vi "Login.vi"() -> ()   [LabVIEW 2020]
uses:
  Global1.vi
panel:
  in  "联机模式":enum16{"单机", "追溯"}(ring)
  in  "密码":string
  in  "账号":string
  in  "确定":bool
  # "锁卡及精密定位圈压装台"
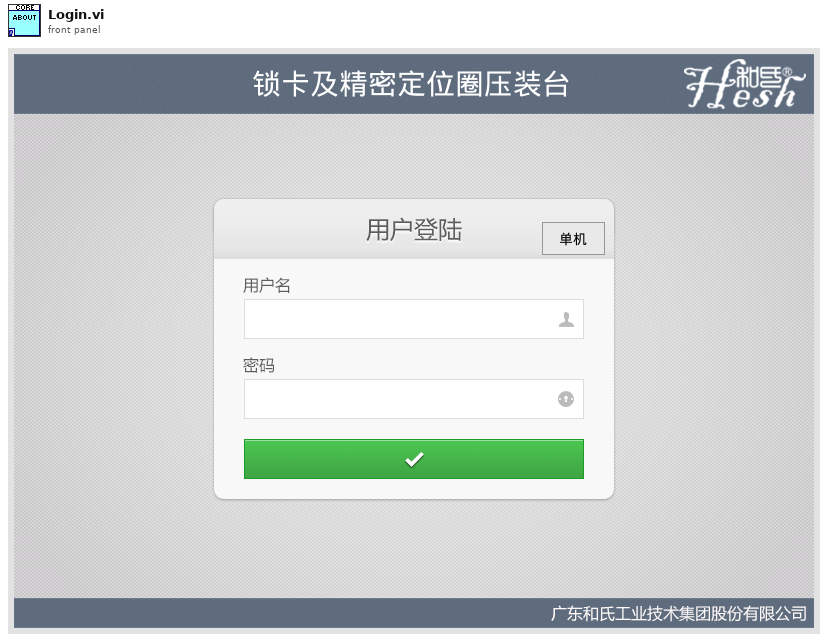
[diagram p1: front panel]
types:
  T1 = enum32{"Invalid", "Standard", "Closed", "Hidden", "Minimized", "Maximized"}
  T2 = cluster{"data[0]":string, "data[1]":string, "data[2]":string, "data[3]":string}
  T3 = typedef "eventvkey.ctl" = enum16{"ASCII", "Enter", "Return", "Shift", "Ctrl", "Alt", "Cmd", "Opt", "Caps", "NumLock", "Clear", "Break", "Up", "Down", "Left", "Right", "Insert", "Delete", "Home", "End", "PageUp", "PageDown", "Escape", "Help", "Pause", "ScrollLock", "F1", "F2", "F3", "F4", "F5", "F6", "F7", "F8", "F9", "F10", "F11", "F12", "F13", "F14", "F15", "F16", "F17", "F18", "F19", "F20", "F21", "F22", "F23", "F24", "Play", "VolumeUp", "VolumeDown", "Mute", "Two Byte Char"}
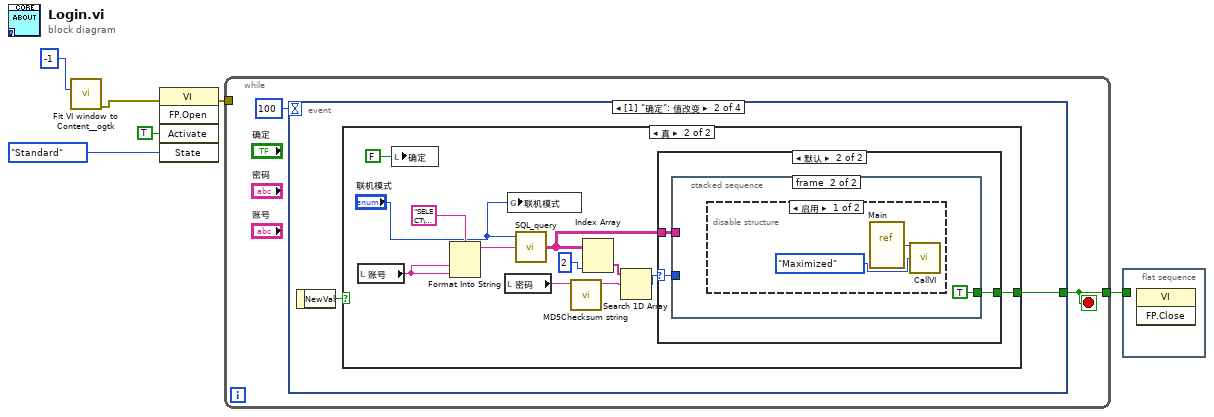
[diagram p0: block diagram]
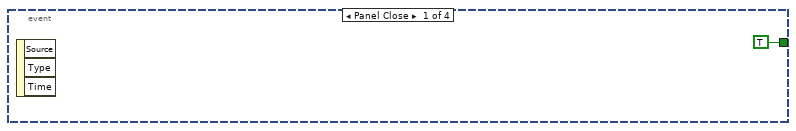
[diagram p2: hidden frame]
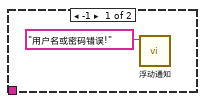
[diagram p4: hidden frame]
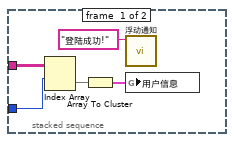
[diagram p5: hidden frame]
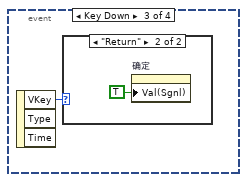
[diagram p7: hidden frame]
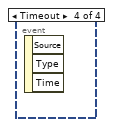
[diagram p9: hidden frame]
diagram:
  n1 = call <userlib>:"Fit VI window to Content__ogtk.vi"("border spacing (2 px)"=-1) -> ("error out"=w1:errorcluster)  [unwired: 5 in, 1 out]
  n2 = invoke class="VI" method="FP.Open"(error in=w1, "Activate"=TRUE ("Activate?"), "State"=T1."Standard") -> (error out=w3:errorcluster)  [unwired: 2 in, 4 out]
  n3 = while {
    tunnel: [w8] -> w6
    tunnel: w3 -> [_]
    stop <- w8 stop-if-true
    n4 = event shown="[1] \"确定\": 值改变" {
      selector: _ -> [_ _ _ _]
      dyn-events: _ -> [_ _ _ _]
      timeout: 100 -> [_ _ _ _]
      tunnel: [TRUE w10 _ _] -> w8
      event Panel Close {
        n5 = event-data() -> ()  [unwired: 4 out]
      }
      event "确定": Value Change {
        n6 = event-data() -> ("NewVal"=w11:bool)  [unwired: 1 out]
        n7 = case shown="真" w11 {
          tunnel: [_ w14] -> w10
          frame False {
          }
          frame True {
            n8 = local read "账号"() -> (w20:string)
            n9 = local write "确定"(FALSE ("确定")) -> ()
            n10 = Format Into String(format string="SELECT\ndbo.[User].USER_EMPLOYEE_ID,\ndbo.[User].USER_NAME,\ndbo.[User].USER_PASSWD,\ndbo.[User].USER_PERMIT\n\nFROM\ndbo.[User]\nWHERE\ndbo.[User].USER_NAME = '%s' \nOR\ndbo.[User].USER_EMPLOYEE_ID = '%s'\n" ("格式字符串"), w20, w20) -> (resulting string=w17:string)  [unwired: 2 in, 1 out]
            n11 = local read "密码"() -> (w21:string)
            n12 = global write "Global1.vi" "联机模式"("联机模式") -> ()
            n13 = call "SQL_query.vi"("SQL query"=w17, "联机模式"="联机模式") -> ("data"=w15:string[][])  [unwired: 1 in, 2 out]
            n14 = call <vilib>:"MD5Checksum string.vi"("Message String"=w21) -> ("MD5 message-digest"=w22:string)  [unwired: 10 in]
            n15 = Index Array(array=w15, index (col)=2 ("禁用的索引 (列)")) -> (element=w19:string[])  [unwired: 1 in]
            n16 = Search 1D Array(1D array=w19, element=w22) -> (index of element=w16:i32)  [unwired: 1 in]
            n17 = case shown="默认" w16 {
              selector: w16 -> [_ w26]
              tunnel: w15 -> [_ w27]
              tunnel: [_ w25] -> w14
              frame -1 {
                n18 = call "浮动通知.vi"("通知内容"="用户名或密码错误!") -> ()  [unwired: 11 in]
              }
              frame Default {
                n19 = stacked-sequence {
                  tunnel: w27 -> [w32 _]
                  tunnel: w26 -> [w31 _]
                  tunnel: [_ TRUE] -> w25
                  frame #0 {
                    n20 = Index Array(array=w32, index (row)=w31) -> (element=w29:string[])  [unwired: 1 in]
                    n21 = Array To Cluster(array=w29) -> (cluster=w28:T2)
                    n22 = call "浮动通知.vi"("通知内容"="登陆成功!") -> ()  [unwired: 11 in]
                    n23 = global write "Global1.vi" "用户信息"(w28) -> ()
                  }
                  frame #1 {
                    n24 = disable-structure shown="启用" {
                      frame Enabled {
                        n25 = vi-ref "Main.vi"() -> (w35:refnum<vi>)
                        n26 = call "CallVI.vi"("VI引用"=w35, "状态"=T1."Maximized") -> ()  [unwired: 11 in, 3 out]
                      }
                      frame Disabled {
                      }
                    }
                  }
                }
              }
            }
          }
        }
      }
      event Key Down {
        n27 = event-data() -> ("VKey"=w36:T3)  [unwired: 3 out]
        n28 = case shown="\"Return\"" w36 {
          frame Default {
          }
          frame "Return" {
            n29 = property on="确定" class="Bool (严格)"("Val(Sgnl)"=TRUE ("值(信号)")) -> ()  [unwired: 2 in, 2 out]
          }
        }
      }
      event Timeout {
        n30 = event-data() -> ()  [unwired: 4 out]
      }
    }
  }
  n31 = flat-sequence {
    tunnel: w6 -> [_]
    frame #0 {
      n32 = invoke class="VI" method="FP.Close"() -> ()  [unwired: 3 in, 3 out]
    }
  }
